vi "interfaceLoop firmwareStateCheck.vi"(8 "error in (no error)":errorcluster, 9 "connectStateRefnum":refnum<data-value>, 11 "Stop":refnum<vi>) -> (0 "error out":errorcluster)   [LabVIEW 2018]
uses:
  <vilib>/Platform/TimedLoop/XDataNode/timing_clust.ctl
  <vilib>/Platform/TimedLoop/XDataNode/nitl_modes.ctl
  <vilib>/Platform/TimedLoop/XDataNode/wakeup.ctl
  <vilib>/Platform/TimedLoop/XDataNode/XDataNode.xnode
  <vilib>/Platform/TimedLoop/XDataNode/XDNodeRunTimeDep.lvlib
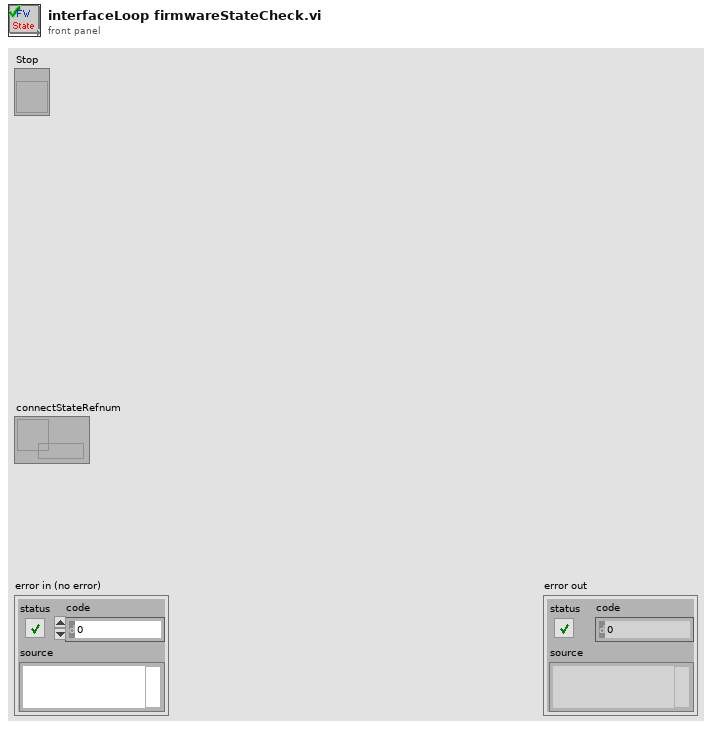
[diagram p1: front panel]
types:
  T1 = typedef "XDNodeRunTimeDep.lvlib/timing_clust.ctl" = cluster{"Expected End [f-1]":u64, "Actual End [f-1]":u64, "Finished Late? [f-1]":bool, "Expected End [i-1]":u64, "Actual End [i-1]":u64, "Finished Late? [i-1]":bool, "Expected Start [i]":u64, "Actual Start [i]":u64, "Expected Start [f]":u64, "Actual Start [f]":u64, "Source Name":string, "Structure Name":string, "Period":i64, "Deadline":i64, "Offset":i64, "Start":i64, "Priority":i32, "Timeout":i32, "Mode":T2, "Wakeup Reason":T3, "Error":errorcluster, "Source Type":string, "Secondary Source Type":string, "Global End Time":u64, "Global Start Time":u64, "Frame Duration":u64, "Iteration Duration":u64, "Assigned CPU":i32, "I/O Scan Engine Mode":u32}
  T2 = typedef "XDNodeRunTimeDep.lvlib/nitl_modes.ctl" = enum32{"No Change", "Process missed periods, maintain original phase", "Discard missed periods, maintain original phase", "Process missed periods, ignore original phase", "Discard missed periods, ignore original phase"}
  T3 = typedef "XDNodeRunTimeDep.lvlib/wakeup.ctl" = enum32{"Normal", "Aborted", "Asynchronous wakeup", "Timing source error", "Timed loop error", "Timeout"}
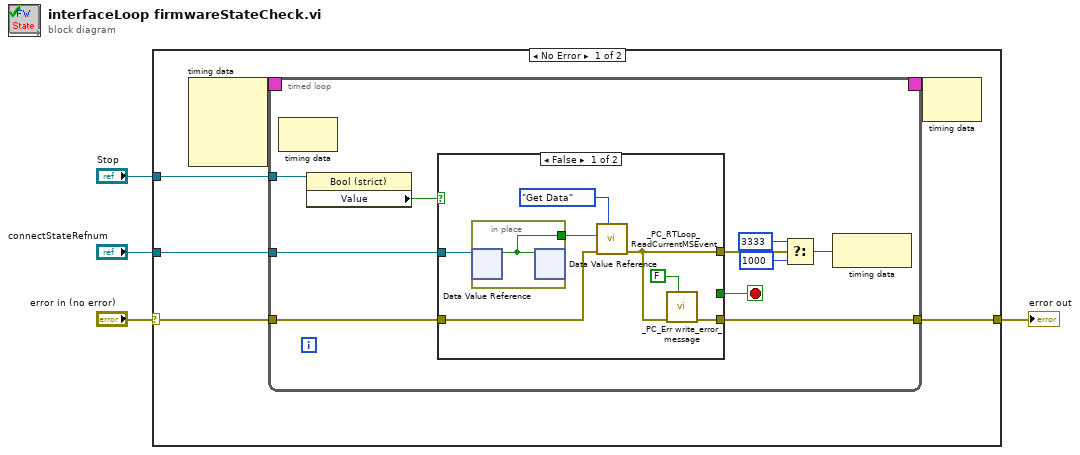
[diagram p0: block diagram]
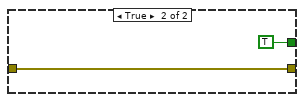
[diagram p2: hidden frame]
diagram:
  n1 = case shown="No Error" "error in (no error)" {
    selector: "error in (no error)" -> [w8 w37]
    tunnel: [w7 w37] -> w1
    tunnel: "Stop" -> [w10 _]
    tunnel: "connectStateRefnum" -> [w9 _]
    frame No Error {
      n2 = node-c288() -> (w6:T1)  [unwired: 4 in]
      n3 = timed-loop {
        tunnel: w10 -> [w20]
        tunnel: w9 -> [w18]
        tunnel: w8 -> [w17]
        tunnel: [w16] -> w7
        timing: w6 -> [_]
        timing-out: [_] -> w5
        stop <- w15 stop-if-true
        n4 = node-c288() -> ()  [unwired: 1 in, 1 out]
        n5 = property class="Bool (strict)"(reference=w20) -> ("Value"=w19:bool)  [unwired: 1 in, 2 out]
        n6 = case shown="False" w19 {
          tunnel: w18 -> [w31 _]
          tunnel: w17 -> [w28 w34]
          tunnel: [w26 w34] -> w16
          tunnel: [_ TRUE] -> w15
          tunnel: [w25 _] -> w14
          frame False {
            n7 = in-place {
              in-place-border: [w32] -> w29
              n8 = in-place-dvr #1(w31) -> (w32:bool)  [unwired: 1 out]
              n9 = in-place-dvr #1(w32) -> ()  [unwired: 2 out]
            }
            n10 = call "_PC_RTLoop_ReadCurrentMSEvent.vi"("Function"=enum16{"Init", "Get Data", "Close"}."Get Data", "error in (no error)"=w28, "connect?"=w29) -> ("error out"=w25:errorcluster)  [unwired: 8 in]
            n11 = call "_PC_Err write_error_message.vi"("show msg( T )"=FALSE, "error in"=w25) -> ("error out"=w26:errorcluster)  [unwired: 9 in]
          }
          frame True {
          }
        }
        n12 = Select(t=i64 3333 ("Period"), s=w14, f=i64 1000 ("Period")) -> (s? t:f=w11:i64)
        n13 = node-c288(w11) -> ()  [unwired: 1 out]
      }
      n14 = node-c288(w5) -> ()  [unwired: 1 out]
    }
    frame Error {
    }
  }
  "error out" <- w1
